vi "Clear-Load Limit Line File.vi"(0 "VISA resource name":refnum<visa-resource-name>, 1 "Upper Limit File Name ( )":path, 5 "Measurement Type (6: Phase Noise)":u16(ring)=6 items=["AM Noise"=1, "Baseband Noise"=2, "Freq/Power"=3, "Spectrum"=4, "Transient"=5, "Phase Noise"=6, "User"=7], 7 "Select Trace (1: 1)":u16(ring)=1 items=["1"=1, "2"=2, "3"=3, "4"=4, "5"=5, "6"=6, "7"=7, "8"=8], 9 "Operation (1: Clear Lower Line)":T1(ring)=enum."Clear Lower Line", 11 "error in (no error)":errorcluster, 12 "Lower Limit File Name ( )":path) -> (4 "VISA resource name out":refnum<visa-resource-name>, 15 "error out":errorcluster)   [LabVIEW 2011, in "Agilent E5052X.lvlib"]
doc: "Clears or loads a selected upper and lower limit line from a specified file location for a specified trace."
uses:
  Agilent E5052X.lvlib
panel:
  # "File Name Settings"
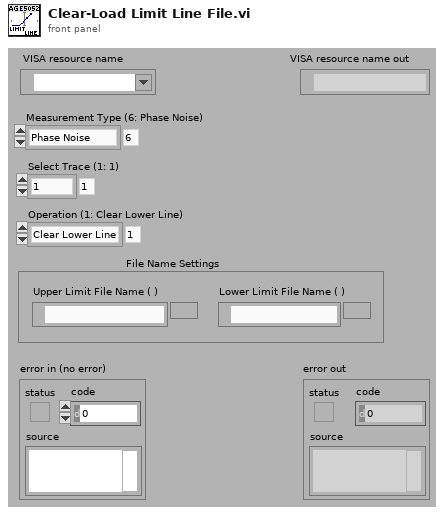
[diagram p1: front panel]
types:
  T1 = enum16{"Load Line", "Clear Lower Line", "Clear Upper Line"}
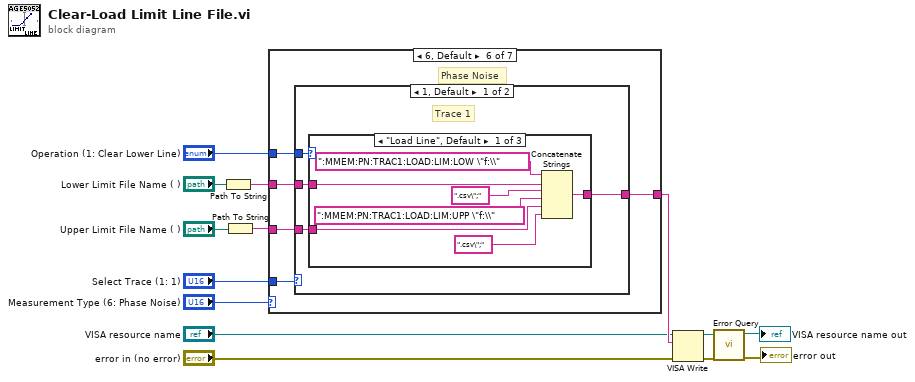
[diagram p0: block diagram]
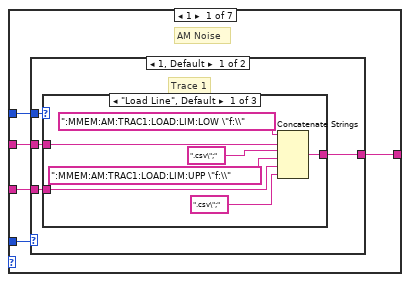
[diagram p2: hidden frame]
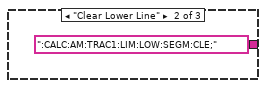
[diagram p3: hidden frame]
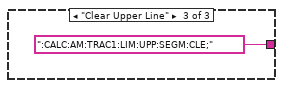
[diagram p4: hidden frame]
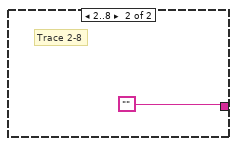
[diagram p5: hidden frame]
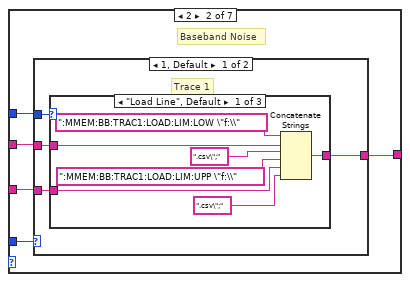
[diagram p6: hidden frame]
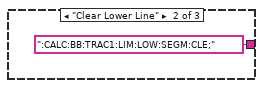
[diagram p7: hidden frame]
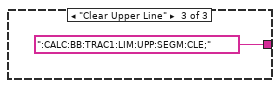
[diagram p8: hidden frame]
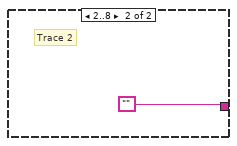
[diagram p9: hidden frame]
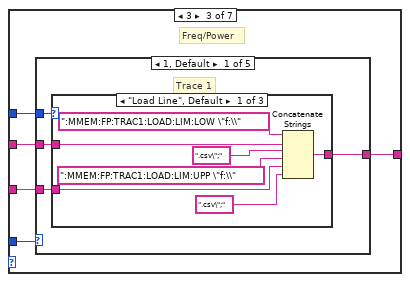
[diagram p10: hidden frame]
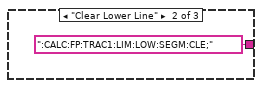
[diagram p11: hidden frame]
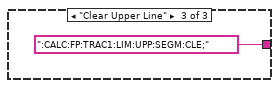
[diagram p12: hidden frame]
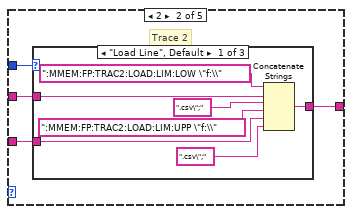
[diagram p13: hidden frame]
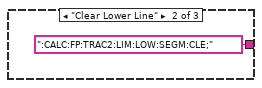
[diagram p14: hidden frame]
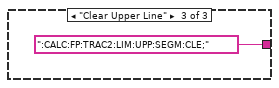
[diagram p15: hidden frame]
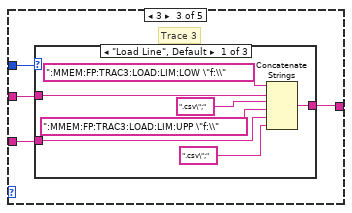
[diagram p16: hidden frame]
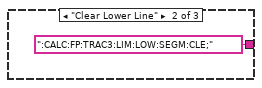
[diagram p17: hidden frame]
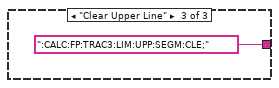
[diagram p18: hidden frame]
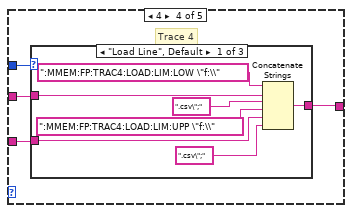
[diagram p19: hidden frame]
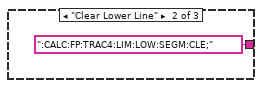
[diagram p20: hidden frame]
diagram:
  n1 = Path To String(path="Lower Limit File Name ( )") -> (string=w3:string)
  n2 = Path To String(path="Upper Limit File Name ( )") -> (string=w1:string)
  n3 = case shown="6, Default" "Measurement Type (6: Phase Noise)" {
    tunnel: "Select Trace (1: 1)" -> [w19 w35 w54 w111 w131 w189 w208]
    tunnel: "Operation (1: Clear Lower Line)" -> [w18 w38 w57 w115 w134 w192 w211]
    tunnel: w3 -> [w17 w37 w56 w114 w133 w191 w210]
    tunnel: w1 -> [w16 w36 w55 w113 w132 w190 w209]
    tunnel: [w15 w34 w53 w112 w130 w188 w207] -> w12
    frame 1 {
      # "AM Noise"
      n4 = case shown="1, Default" w19 {
        tunnel: w18 -> [w23 _]
        tunnel: w17 -> [w22 _]
        tunnel: w16 -> [w21 _]
        tunnel: [w20 ""] -> w15
        frame 1, Default {
          # "Trace 1"
          n5 = case shown="\"Load Line\", Default" w23 {
            tunnel: w22 -> [w29 _ _]
            tunnel: w21 -> [w25 _ _]
            tunnel: [w27 ":CALC:AM:TRAC1:LIM:LOW:SEGM:CLE;" ":CALC:AM:TRAC1:LIM:UPP:SEGM:CLE;"] -> w20
            frame "Load Line", Default {
              n6 = Concatenate Strings(":MMEM:AM:TRAC1:LOAD:LIM:LOW \"f:\\", w29, ".csv\";" ("string"), ":MMEM:AM:TRAC1:LOAD:LIM:UPP \"f:\\", w25, ".csv\";" ("string")) -> (w27:string)
            }
            frame "Clear Lower Line" {
            }
            frame "Clear Upper Line" {
            }
          }
        }
        frame 2..8 {
          # "Trace 2-8"
        }
      }
    }
    frame 2 {
      # "Baseband Noise"
      n7 = case shown="1, Default" w35 {
        tunnel: w38 -> [w42 _]
        tunnel: w37 -> [w41 _]
        tunnel: w36 -> [w40 _]
        tunnel: [w39 ""] -> w34
        frame 1, Default {
          # "Trace 1"
          n8 = case shown="\"Load Line\", Default" w42 {
            tunnel: w41 -> [w48 _ _]
            tunnel: w40 -> [w44 _ _]
            tunnel: [w46 ":CALC:BB:TRAC1:LIM:LOW:SEGM:CLE;" ":CALC:BB:TRAC1:LIM:UPP:SEGM:CLE;"] -> w39
            frame "Load Line", Default {
              n9 = Concatenate Strings(":MMEM:BB:TRAC1:LOAD:LIM:LOW \"f:\\", w48, ".csv\";" ("string"), ":MMEM:BB:TRAC1:LOAD:LIM:UPP \"f:\\", w44, ".csv\";" ("string")) -> (w46:string)
            }
            frame "Clear Lower Line" {
            }
            frame "Clear Upper Line" {
            }
          }
        }
        frame 2..8 {
          # "Trace 2"
        }
      }
    }
    frame 3 {
      # "Freq/Power"
      n10 = case shown="1, Default" w54 {
        tunnel: w57 -> [w61 w73 w87 w100 _]
        tunnel: w56 -> [w60 w72 w86 w99 _]
        tunnel: w55 -> [w59 w71 w85 w98 _]
        tunnel: [w58 w74 w84 w97 ""] -> w53
        frame 1, Default {
          # "Trace 1"
          n11 = case shown="\"Load Line\", Default" w61 {
            tunnel: w60 -> [w67 _ _]
            tunnel: w59 -> [w63 _ _]
            tunnel: [w65 ":CALC:FP:TRAC1:LIM:LOW:SEGM:CLE;" ":CALC:FP:TRAC1:LIM:UPP:SEGM:CLE;"] -> w58
            frame "Load Line", Default {
              n12 = Concatenate Strings(":MMEM:FP:TRAC1:LOAD:LIM:LOW \"f:\\", w67, ".csv\";" ("string"), ":MMEM:FP:TRAC1:LOAD:LIM:UPP \"f:\\", w63, ".csv\";" ("string")) -> (w65:string)
            }
            frame "Clear Lower Line" {
            }
            frame "Clear Upper Line" {
            }
          }
        }
        frame 2 {
          # "Trace 2"
          n13 = case shown="\"Load Line\", Default" w73 {
            tunnel: w72 -> [w80 _ _]
            tunnel: w71 -> [w76 _ _]
            tunnel: [w78 ":CALC:FP:TRAC2:LIM:LOW:SEGM:CLE;" ":CALC:FP:TRAC2:LIM:UPP:SEGM:CLE;"] -> w74
            frame "Load Line", Default {
              n14 = Concatenate Strings(":MMEM:FP:TRAC2:LOAD:LIM:LOW \"f:\\", w80, ".csv\";" ("string"), ":MMEM:FP:TRAC2:LOAD:LIM:UPP \"f:\\", w76, ".csv\";" ("string")) -> (w78:string)
            }
            frame "Clear Lower Line" {
            }
            frame "Clear Upper Line" {
            }
          }
        }
        frame 3 {
          # "Trace 3"
          n15 = case shown="\"Load Line\", Default" w87 {
            tunnel: w86 -> [w93 _ _]
            tunnel: w85 -> [w89 _ _]
            tunnel: [w91 ":CALC:FP:TRAC3:LIM:LOW:SEGM:CLE;" ":CALC:FP:TRAC3:LIM:UPP:SEGM:CLE;"] -> w84
            frame "Load Line", Default {
              n16 = Concatenate Strings(":MMEM:FP:TRAC3:LOAD:LIM:LOW \"f:\\", w93, ".csv\";" ("string"), ":MMEM:FP:TRAC3:LOAD:LIM:UPP \"f:\\", w89, ".csv\";" ("string")) -> (w91:string)
            }
            frame "Clear Lower Line" {
            }
            frame "Clear Upper Line" {
            }
          }
        }
        frame 4 {
          # "Trace 4"
          n17 = case shown="\"Load Line\", Default" w100 {
            tunnel: w99 -> [w106 _ _]
            tunnel: w98 -> [w102 _ _]
            tunnel: [w104 ":CALC:FP:TRAC4:LIM:LOW:SEGM:CLE;" ":CALC:FP:TRAC4:LIM:UPP:SEGM:CLE;"] -> w97
            frame "Load Line", Default {
              n18 = Concatenate Strings(":MMEM:FP:TRAC4:LOAD:LIM:LOW \"f:\\", w106, ".csv\";" ("string"), ":MMEM:FP:TRAC4:LOAD:LIM:UPP \"f:\\", w102, ".csv\";" ("string")) -> (w104:string)
            }
            frame "Clear Lower Line" {
            }
            frame "Clear Upper Line" {
            }
          }
        }
        frame 5..8 {
          # "Trace 5-8"
        }
      }
    }
    frame 4 {
      # "Spectrum"
      n19 = case shown="1, Default" w111 {
        tunnel: w115 -> [w119 _]
        tunnel: w114 -> [w118 _]
        tunnel: w113 -> [w117 _]
        tunnel: [w116 ""] -> w112
        frame 1, Default {
          # "Trace 1"
          n20 = case shown="\"Load Line\", Default" w119 {
            tunnel: w118 -> [w125 _ _]
            tunnel: w117 -> [w121 _ _]
            tunnel: [w123 ":CALC:SP:TRAC1:LIM:LOW:SEGM:CLE;" ":CALC:SP:TRAC1:LIM:UPP:SEGM:CLE;"] -> w116
            frame "Load Line", Default {
              n21 = Concatenate Strings(":MMEM:SP:TRAC1:LOAD:LIM:LOW \"f:\\", w125, ".csv\";" ("string"), ":MMEM:SP:TRAC1:LOAD:LIM:UPP \"f:\\", w121, ".csv\";" ("string")) -> (w123:string)
            }
            frame "Clear Lower Line" {
            }
            frame "Clear Upper Line" {
            }
          }
        }
        frame 2..8 {
          # "Trace 2-8"
        }
      }
    }
    frame 5 {
      # "Transient"
      n22 = case shown="1, Default" w131 {
        tunnel: w134 -> [w138 w150 w164 w177 _]
        tunnel: w133 -> [w137 w149 w163 w176 _]
        tunnel: w132 -> [w136 w148 w162 w175 _]
        tunnel: [w135 w151 w161 w174 ""] -> w130
        frame 1, Default {
          # "Trace 1"
          n23 = case shown="\"Load Line\", Default" w138 {
            tunnel: w137 -> [w144 _ _]
            tunnel: w136 -> [w140 _ _]
            tunnel: [w142 ":CALC:TR:TRAC1:LIM:LOW:SEGM:CLE;" ":CALC:TR:TRAC1:LIM:UPP:SEGM:CLE;"] -> w135
            frame "Load Line", Default {
              n24 = Concatenate Strings(":MMEM:TR:TRAC1:LOAD:LIM:LOW \"f:/", w144, ".csv\";" ("string"), ":MMEM:TR:TRAC1:LOAD:LIM:UPP \"f:/", w140, ".csv\";" ("string")) -> (w142:string)
            }
            frame "Clear Lower Line" {
            }
            frame "Clear Upper Line" {
            }
          }
        }
        frame 2 {
          # "Trace 2"
          n25 = case shown="\"Load Line\", Default" w150 {
            tunnel: w149 -> [w157 _ _]
            tunnel: w148 -> [w153 _ _]
            tunnel: [w155 ":CALC:TR:TRAC2:LIM:LOW:SEGM:CLE;" ":CALC:TR:TRAC2:LIM:UPP:SEGM:CLE;"] -> w151
            frame "Load Line", Default {
              n26 = Concatenate Strings(":MMEM:TR:TRAC2:LOAD:LIM:LOW \"f:\\", w157, ".csv\";" ("string"), ":MMEM:TR:TRAC2:LOAD:LIM:UPP \"f:\\", w153, ".csv\";" ("string")) -> (w155:string)
            }
            frame "Clear Lower Line" {
            }
            frame "Clear Upper Line" {
            }
          }
        }
        frame 3 {
          # "Trace 3"
          n27 = case shown="\"Load Line\", Default" w164 {
            tunnel: w163 -> [w170 _ _]
            tunnel: w162 -> [w166 _ _]
            tunnel: [w168 ":CALC:TR:TRAC3:LIM:LOW:SEGM:CLE;" ":CALC:TR:TRAC3:LIM:UPP:SEGM:CLE;"] -> w161
            frame "Load Line", Default {
              n28 = Concatenate Strings(":MMEM:TR:TRAC3:LOAD:LIM:LOW \"f:\\", w170, ".csv\";" ("string"), ":MMEM:TR:TRAC3:LOAD:LIM:UPP \"f:\\", w166, ".csv\";" ("string")) -> (w168:string)
            }
            frame "Clear Lower Line" {
            }
            frame "Clear Upper Line" {
            }
          }
        }
        frame 4 {
          # "Trace 4"
          n29 = case shown="\"Load Line\", Default" w177 {
            tunnel: w176 -> [w183 _ _]
            tunnel: w175 -> [w179 _ _]
            tunnel: [w181 ":CALC:TR:TRAC4:LIM:LOW:SEGM:CLE;" ":CALC:TR:TRAC4:LIM:UPP:SEGM:CLE;"] -> w174
            frame "Load Line", Default {
              n30 = Concatenate Strings(":MMEM:TR:TRAC4:LOAD:LIM:LOW \"f:\\", w183, ".csv\";" ("string"), ":MMEM:TR:TRAC4:LOAD:LIM:UPP \"f:\\", w179, ".csv\";" ("string")) -> (w181:string)
            }
            frame "Clear Lower Line" {
            }
            frame "Clear Upper Line" {
            }
          }
        }
        frame 5..8 {
          # "Trace 5-8"
        }
      }
    }
    frame 6, Default {
      # "Phase Noise"
      n31 = case shown="1, Default" w189 {
        tunnel: w192 -> [w196 _]
        tunnel: w191 -> [w195 _]
        tunnel: w190 -> [w194 _]
        tunnel: [w193 ""] -> w188
        frame 1, Default {
          # "Trace 1"
          n32 = case shown="\"Load Line\", Default" w196 {
            tunnel: w195 -> [w202 _ _]
            tunnel: w194 -> [w198 _ _]
            tunnel: [w200 ":CALC:PN:TRAC1:LIM:LOW:SEGM:CLE;" ":CALC:PN:TRAC1:LIM:UPP:SEGM:CLE;"] -> w193
            frame "Load Line", Default {
              n33 = Concatenate Strings(":MMEM:PN:TRAC1:LOAD:LIM:LOW \"f:\\", w202, ".csv\";" ("string"), ":MMEM:PN:TRAC1:LOAD:LIM:UPP \"f:\\", w198, ".csv\";" ("string")) -> (w200:string)
            }
            frame "Clear Lower Line" {
            }
            frame "Clear Upper Line" {
            }
          }
        }
        frame 2..8 {
          # "Trace 2-8"
        }
      }
    }
    frame 7 {
      # "User"
      n34 = case shown="1, Default" w208 {
        tunnel: w211 -> [w215 w227 w241 w254 w267 w280 w293 w306]
        tunnel: w210 -> [w214 w226 w240 w253 w266 w279 w292 w305]
        tunnel: w209 -> [w213 w225 w239 w252 w265 w278 w291 w304]
        tunnel: [w212 w228 w238 w251 w264 w277 w290 w303] -> w207
        frame 1, Default {
          # "Trace 1"
          n35 = case shown="\"Load Line\", Default" w215 {
            tunnel: w214 -> [w221 _ _]
            tunnel: w213 -> [w217 _ _]
            tunnel: [w219 ":CALC:USER:TRAC1:LIM:LOW:SEGM:CLE;" ":CALC:USER:TRAC1:LIM:UPP:SEGM:CLE;"] -> w212
            frame "Load Line", Default {
              n36 = Concatenate Strings(":MMEM:USER:TRAC1:LOAD:LIM:LOW \"f:\\", w221, ".csv\";" ("string"), ":MMEM:USER:TRAC1:LOAD:LIM:UPP \"f:\\", w217, ".csv\";" ("string")) -> (w219:string)
            }
            frame "Clear Lower Line" {
            }
            frame "Clear Upper Line" {
            }
          }
        }
        frame 2 {
          # "Trace 2"
          n37 = case shown="\"Load Line\", Default" w227 {
            tunnel: w226 -> [w234 _ _]
            tunnel: w225 -> [w230 _ _]
            tunnel: [w232 ":CALC:USER:TRAC2:LIM:LOW:SEGM:CLE;" ":CALC:USER:TRAC2:LIM:UPP:SEGM:CLE;"] -> w228
            frame "Load Line", Default {
              n38 = Concatenate Strings(":MMEM:USER:TRAC2:LOAD:LIM:LOW \"f:\\", w234, ".csv\";" ("string"), ":MMEM:USER:TRAC2:LOAD:LIM:UPP \"f:\\", w230, ".csv\";" ("string")) -> (w232:string)
            }
            frame "Clear Lower Line" {
            }
            frame "Clear Upper Line" {
            }
          }
        }
        frame 3 {
          # "Trace 3"
          n39 = case shown="\"Load Line\", Default" w241 {
            tunnel: w240 -> [w247 _ _]
            tunnel: w239 -> [w243 _ _]
            tunnel: [w245 ":CALC:USER:TRAC3:LIM:LOW:SEGM:CLE;" ":CALC:USER:TRAC3:LIM:UPP:SEGM:CLE;"] -> w238
            frame "Load Line", Default {
              n40 = Concatenate Strings(":MMEM:USER:TRAC3:LOAD:LIM:LOW \"f:\\", w247, ".csv\";" ("string"), ":MMEM:USER:TRAC3:LOAD:LIM:UPP \"f:\\", w243, ".csv\";" ("string")) -> (w245:string)
            }
            frame "Clear Lower Line" {
            }
            frame "Clear Upper Line" {
            }
          }
        }
        frame 4 {
          # "Trace 4"
          n41 = case shown="\"Load Line\", Default" w254 {
            tunnel: w253 -> [w260 _ _]
            tunnel: w252 -> [w256 _ _]
            tunnel: [w258 ":CALC:USER:TRAC4:LIM:LOW:SEGM:CLE;" ":CALC:USER:TRAC4:LIM:UPP:SEGM:CLE;"] -> w251
            frame "Load Line", Default {
              n42 = Concatenate Strings(":MMEM:USER:TRAC4:LOAD:LIM:LOW \"f:\\", w260, ".csv\";" ("string"), ":MMEM:USER:TRAC4:LOAD:LIM:UPP \"f:\\", w256, ".csv\";" ("string")) -> (w258:string)
            }
            frame "Clear Lower Line" {
            }
            frame "Clear Upper Line" {
            }
          }
        }
        frame 5 {
          # "Trace 5"
          n43 = case shown="\"Load Line\", Default" w267 {
            tunnel: w266 -> [w273 _ _]
            tunnel: w265 -> [w269 _ _]
            tunnel: [w271 ":CALC:USER:TRAC5:LIM:LOW:SEGM:CLE;" ":CALC:USER:TRAC5:LIM:UPP:SEGM:CLE;"] -> w264
            frame "Load Line", Default {
              n44 = Concatenate Strings(":MMEM:USER:TRAC5:LOAD:LIM:LOW \"f:\\", w273, ".csv\";" ("string"), ":MMEM:USER:TRAC5:LOAD:LIM:UPP \"f:\\", w269, ".csv\";" ("string")) -> (w271:string)
            }
            frame "Clear Lower Line" {
            }
            frame "Clear Upper Line" {
            }
          }
        }
        frame 6 {
          # "Trace 6"
          n45 = case shown="\"Load Line\", Default" w280 {
            tunnel: w279 -> [w286 _ _]
            tunnel: w278 -> [w282 _ _]
            tunnel: [w284 ":CALC:USER:TRAC6:LIM:LOW:SEGM:CLE;" ":CALC:USER:TRAC6:LIM:UPP:SEGM:CLE;"] -> w277
            frame "Load Line", Default {
              n46 = Concatenate Strings(":MMEM:USER:TRAC6:LOAD:LIM:LOW \"f:\\", w286, ".csv\";" ("string"), ":MMEM:USER:TRAC6:LOAD:LIM:UPP \"f:\\", w282, ".csv\";" ("string")) -> (w284:string)
            }
            frame "Clear Lower Line" {
            }
            frame "Clear Upper Line" {
            }
          }
        }
        frame 7 {
          # "Trace 7"
          n47 = case shown="\"Load Line\", Default" w293 {
            tunnel: w292 -> [w299 _ _]
            tunnel: w291 -> [w295 _ _]
            tunnel: [w297 ":CALC:USER:TRAC7:LIM:LOW:SEGM:CLE;" ":CALC:USER:TRAC7:LIM:UPP:SEGM:CLE;"] -> w290
            frame "Load Line", Default {
              n48 = Concatenate Strings(":MMEM:USER:TRAC7:LOAD:LIM:LOW \"f:\\", w299, ".csv\";" ("string"), ":MMEM:USER:TRAC7:LOAD:LIM:UPP \"f:\\", w295, ".csv\";" ("string")) -> (w297:string)
            }
            frame "Clear Lower Line" {
            }
            frame "Clear Upper Line" {
            }
          }
        }
        frame 8 {
          # "Trace 8"
          n49 = case shown="\"Load Line\", Default" w306 {
            tunnel: w305 -> [w312 _ _]
            tunnel: w304 -> [w308 _ _]
            tunnel: [w310 ":CALC:USER:TRAC8:LIM:LOW:SEGM:CLE;" ":CALC:USER:TRAC8:LIM:UPP:SEGM:CLE;"] -> w303
            frame "Load Line", Default {
              n50 = Concatenate Strings(":MMEM:USER:TRAC8:LOAD:LIM:LOW \"f:\\", w312, ".csv\";" ("string"), ":MMEM:USER:TRAC8:LOAD:LIM:UPP \"f:\\", w308, ".csv\";" ("string")) -> (w310:string)
            }
            frame "Clear Lower Line" {
            }
            frame "Clear Upper Line" {
            }
          }
        }
      }
    }
  }
  n51 = VISA Write(VISA resource name="VISA resource name", write buffer=w12, error in (no error)="error in (no error)") -> (VISA resource name out=w11:refnum<visa-resource-name>, error out=w10:errorcluster)  [unwired: 1 out]
  n52 = call "Error Query.vi"("error in (no error)"=w10, "VISA resource name"=w11) -> ("error out"=→"error out":errorcluster, "VISA resource name out"=→"VISA resource name out":refnum<visa-resource-name>)  [unwired: 6 in, 2 out]
